vi "StartVideo Begin.vi"(8 "error in (no error)":errorcluster, 9 "Script":string, 10 "Media Source":string, 11 "VLC Variables In in":T1) -> (0 "error out":errorcluster, 3 "VLC Variables In out":T1)   [LabVIEW 2012]
uses:
  Controls-Webcam/VLC Var.ctl
  Program Files (x86)/VideoLAN/VLC/libvlc.dll
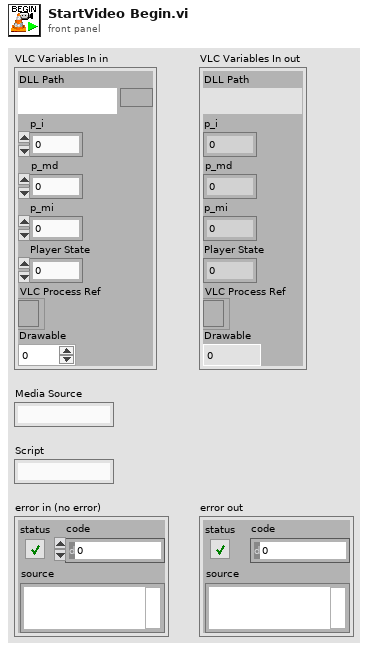
[diagram p1: front panel]
types:
  T1 = typedef "VLC Var.ctl" = cluster{"DLL Path":path, "p_i":i32, "p_md":i32, "p_mi":i32, "Player State":i32, "VLC Process Ref":refnum<k24>, "Drawable":i32}
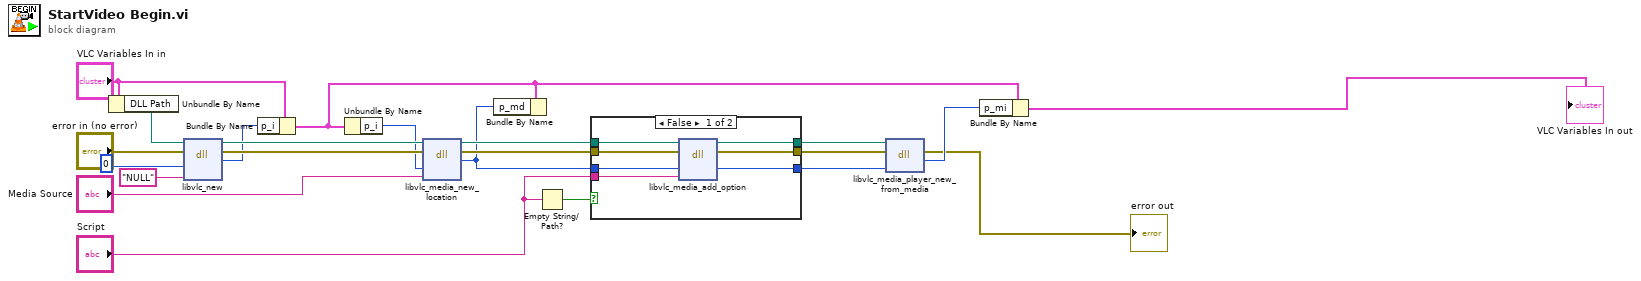
[diagram p0: block diagram]
diagram:
  n1 = Unbundle By Name("VLC Variables In in") -> ("DLL Path"=w20:path)
  n2 = dll-call lib="C:/Program Files (x86)/VideoLAN/VLC/libvlc.dll" fn="libvlc_new"(path in=w20, error in="error in (no error)", "argc"=i16 0, "argv"="NULL") -> (path out=w13:path, error out=w5:errorcluster, "return type"=w3:i32)  [unwired: 3 in]
  n3 = Bundle By Name(cluster="VLC Variables In in", "p_i"=w3) -> (w17:T1)
  n4 = Unbundle By Name(w17) -> ("p_i"=w2:i32)
  n5 = dll-call lib="C:/Program Files (x86)/VideoLAN/VLC/libvlc.dll" fn="libvlc_media_new_location"(path in=w13, error in=w5, "p_instance"=w2, "path"="Media Source") -> (path out=w14:path, error out=w9:errorcluster, "return type"=w7:i32)  [unwired: 3 in]
  n6 = Bundle By Name(cluster=w17, "p_md"=w7) -> ()  [unwired: 1 out]
  n7 = Empty String/Path?(string/path="Script") -> (empty?=w12:bool)
  n8 = case shown="False" w12 {
    tunnel: w9 -> [w28 w31]
    tunnel: w7 -> [w27 w30]
    tunnel: [w26 w30] -> w8
    tunnel: [w25 w31] -> w10
    tunnel: "Script" -> [w24 _]
    tunnel: w14 -> [w23 w29]
    tunnel: [w23 w29] -> w11
    frame False {
      n9 = dll-call lib="C:/Program Files (x86)/VideoLAN/VLC/libvlc.dll" fn="libvlc_media_add_option"(error in=w28, "p_md"=w27, "ppsz_options"=w24) -> (error out=w25:errorcluster, "p_md"=w26:i32)  [unwired: 4 in, 1 out]
    }
    frame True {
    }
  }
  n10 = dll-call lib="C:/Program Files (x86)/VideoLAN/VLC/libvlc.dll" fn="libvlc_media_player_new_from_media"(path in=w11, error in=w10, "p_md"=w8) -> (error out=→"error out":errorcluster, "return type"=w22:i32)  [unwired: 2 in, 1 out]
  n11 = Bundle By Name(cluster=w17, "p_mi"=w22) -> (→"VLC Variables In out":T1)
